vi "sc5511a_get_device_status.vi"(0 "deviceHandle":u32 format="%.0x", 5 "error in":errorcluster) -> (14 "deviceHandle":u32 format="%.0x", 16 "Device Status":T1 {"PLL Status"."Lo2 PLL" items=["Unlocked", "Locked"]; "PLL Status"."Clk 10 PLL" items=["Unlocked", "Locked"]; "PLL Status"."Ref Clk PLL" items=["NOT Locked", "Locked"]; "PLL Status"."Crs assist PLL" items=["NOT Locked", "Locked"]; "PLL Status"."Crs Ref PLL" items=["NOT Locked", "Locked"]; "PLL Status"."Fine PLL" items=["NOT Locked", "Locked"]; "PLL Status"."Crs PLL" items=["NOT Locked", "Locked"]; "PLL Status"."Sum PLL" items=["NOT Locked", "Locked"]; "List Mode Config"."Trigger Out Behavior" items=["Trigger On Step", "Trigger On Cycle"]; "List Mode Config"."Trigger Out State" items=["Trigger Out Disable", "Trigger Out Enable"]; "List Mode Config"."Return to Start" items=["Stop at End", "Return to Start"]; "List Mode Config"."HW Trigger Mode" items=["Start/Stop", "Step"]; "List Mode Config"."Trigger Source" items=["Software", "Hardware"]; "List Mode Config"."Shape" items=["Sawtooth", "Triangle"]; "List Mode Config"."Direction" items=["Low to High", "High to Low"]; "List Mode Config"."List/SSS" items=["List", "Start/Stop/Step"]; "Operate Status"."Harmonic SS" items=["Enable", "Disable"]; "Operate Status"."Loop Gain" items=["Normal", "Low"]; "Operate Status"."RFOutState" items=["Disable", "Enable"]; "Operate Status"."ExtRefDetected" items=["No Ref available", "Ext Ref detected"]; "Operate Status"."RF2 Standby" items=["Disabled", "Enabled"]; "Operate Status"."AlcMode" items=["ALC closed", "ALC opened"]; "Operate Status"."AutoPwrLevel" items=["Disabled", "Enabled"]; "Operate Status"."OverTempStatus" items=["Normal", "OverTemp"]; "Operate Status"."RF Mode" items=["Fixed Tone", "List Mode"]; "Operate Status"."ListRuning" items=["Not active", "Active"]; "Operate Status"."RefOutSelect" items=["10MHz enabled", "100MHz enabled"]; "Operate Status"."Lock Mode" items=["Harmonic Loop", "fracN Loop"]; "Operate Status"."RF1 Standby" items=["Stdby disabled", "Stdby enabled"]; "Operate Status"."Device Accessed" items=["Not accessed", "accessed"]; "Operate Status"."Ref Lock Enable" items=["Lock disabled", "Lock enabled"]}, 19 "error out":errorcluster)   [LabVIEW 2010]
uses:
  sc5511a.dll
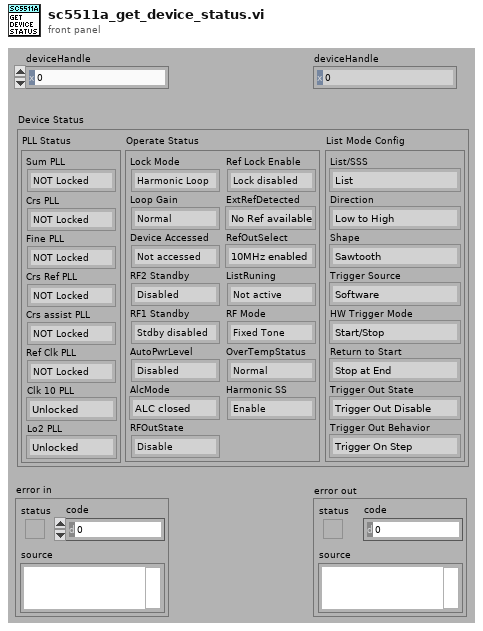
[diagram p1: front panel]
types:
  T1 = cluster{"List Mode Config":cluster{"List/SSS":u8, "Direction":u8, "Shape":u8, "Trigger Source":u8, "HW Trigger Mode":u8, "Return to Start":u8, "Trigger Out State":u8, "Trigger Out Behavior":u8}, "Operate Status":cluster{"Lock Mode":u8, "Loop Gain":u8, "Device Accessed":u8, "RF2 Standby":u8, "RF1 Standby":u8, "AutoPwrLevel":u8, "AlcMode":u8, "RFOutState":u8, "Ref Lock Enable":u8, "ExtRefDetected":u8, "RefOutSelect":u8, "ListRuning":u8, "RF Mode":u8, "OverTempStatus":u8, "Harmonic SS":u8}, "PLL Status":cluster{"Sum PLL":u8, "Crs PLL":u8, "Fine PLL":u8, "Crs Ref PLL":u8, "Crs assist PLL":u8, "Ref Clk PLL":u8, "Clk 10 PLL":u8, "Lo2 PLL":u8}}
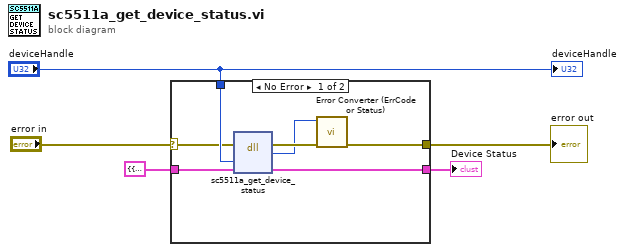
[diagram p0: block diagram]
diagram:
  n1 = case shown="No Error" "error in" {
    selector: "error in" -> [w6 w14]
    tunnel: [w12 w14] -> w4
    tunnel: "deviceHandle" -> [w9 _]
    tunnel: T1 {"List Mode Config"={"List/SSS"=0, "Direction"=0, "Shape"=0, "Trigger Source"=0, "HW Trigger Mode"=0, "Return to Start"=0, "Trigger Out State"=0, "Trigger Out Behavior"=0}, "Operate Status"={"Lock Mode"=0, "Loop Gain"=0, "Device Accessed"=0, "RF2 Standby"=0, "RF1 Standby"=0, "AutoPwrLevel"=0, "AlcMode"=0, "RFOutState"=0, "Ref Lock Enable"=0, "ExtRefDetected"=0, "RefOutSelect"=0, "ListRuning"=0, "RF Mode"=0, "OverTempStatus"=0, "Harmonic SS"=0}, "PLL Status"={"Sum PLL"=0, "Crs PLL"=0, "Fine PLL"=0, "Crs Ref PLL"=0, "Crs assist PLL"=0, "Ref Clk PLL"=0, "Clk 10 PLL"=0, "Lo2 PLL"=0}} ("Device Status 2") -> [w8 w13]
    tunnel: [w7 w13] -> w2
    frame No Error {
      n2 = dll-call lib="sc5511a.dll" fn="sc5511a_get_device_status"(error in=w6, "deviceHandle"=w9, "Device Status"=w8) -> (error out=w11:errorcluster, "return type"=w10:i32, "Device Status"=w7:T1)  [unwired: 3 in, 1 out]
      n3 = call "Error Converter (ErrCode or Status).vi"("error in (no error)"=w11, "error code"=w10) -> ("error out"=w12:errorcluster)  [unwired: 9 in]
    }
    frame Error {
    }
  }
  "error out" <- w4
  "Device Status" <- w2
  "deviceHandle" <- "deviceHandle"
